vi "Date Time Rec to Timestamp.vi"(0 "date time record":T1) -> (1 "timestamp object":timestamp format="%<%m/%d/%Y %H:%M:%S>T", 2 "timestamp seconds":dbl)   [LabVIEW 2010]
doc: "Convert a Date and Time Record to a Timestamp Object and \"seconds since 1904\", without DST adjustments. Removing the DST adjustment causes the date time record hour to match the Timestamp Object hour."
uses:
  <vilib>/Utility/miscctls.llb/LVDateTimeRec.ctl
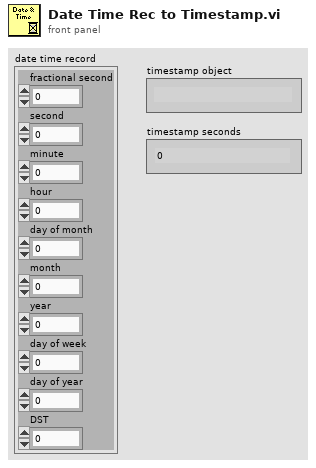
[diagram p1: front panel]
types:
  T1 = typedef "LVDateTimeRec.ctl" = cluster{"fractional second":dbl, "second":i32, "minute":i32, "hour":i32, "day of month":i32, "month":i32, "year":i32, "day of week":i32, "day of year":i32, "DST":i32}
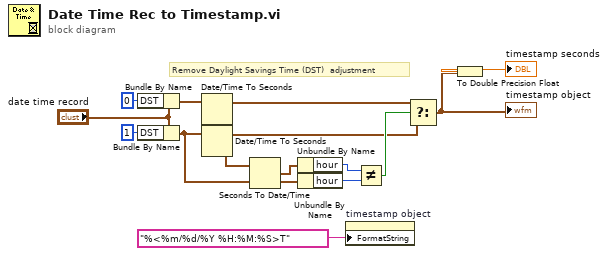
[diagram p0: block diagram]
diagram:
  # "Remove Daylight Savings Time (DST)  adjustment"
  n1 = Bundle By Name(cluster="date time record", "DST"=0) -> (w4:T1)
  n2 = Bundle By Name(cluster="date time record", "DST"=1) -> (w3:T1)
  n3 = Date/Time To Seconds(2:w4) -> (0:w9:timestamp)  [unwired: 1 in]
  n4 = Date/Time To Seconds(2:w3) -> (0:w8:timestamp)  [unwired: 1 in]
  n5 = Seconds To Date/Time(time stamp (now)=w8) -> (date time rec=w12:T1)  [unwired: 1 in]
  n6 = Unbundle By Name(w12) -> ("hour"=w11:i32)
  n7 = Unbundle By Name(w3) -> ("hour"=w2:i32)
  n8 = property on="timestamp object" class="AbsTime (strict)"("FormatString"="%<%m/%d/%Y %H:%M:%S>T" ("delimiters (\\s,\\t,\\r,\\n)")) -> ()  [unwired: 2 in, 2 out]
  n9 = Not Equal?(x=w11, y=w2) -> (x != y?=w10:bool)
  n10 = Select(t=w9, s=w10, f=w8) -> (s? t:f=w7:timestamp)
  "timestamp object" <- w7
  n11 = To Double Precision Float(number=w7) -> (double precision float=→"timestamp seconds":dbl)
